vi "CFG Parse Registry Instructions.vi"(0 "Special Instructions":string, 1 "Section":string) -> (4 "Subkey":string, 8 "Registry Item":bool)   [LabVIEW 2012]
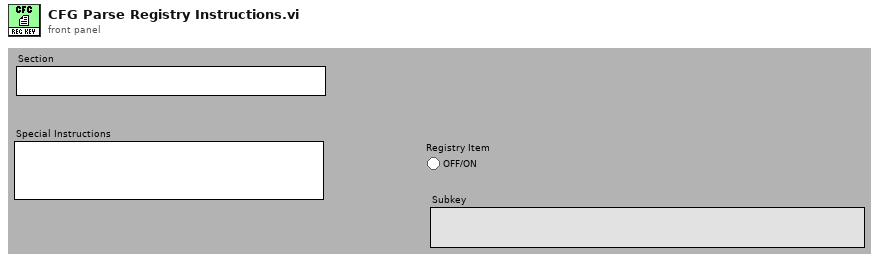
[diagram p1: front panel]
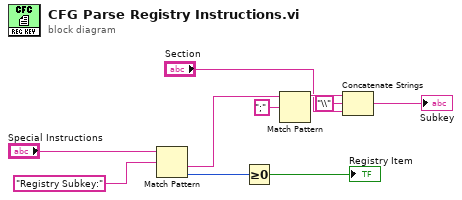
[diagram p0: block diagram]
diagram:
  n1 = Match Pattern(string="Special Instructions", regular expression="Registry Subkey:") -> (after substring=w6:string, offset past match=w9:i32)  [unwired: 3 out]
  n2 = Greater Or Equal To 0?(x=w9) -> (x >= 0?=→"Registry Item":bool)
  n3 = Match Pattern(string=w6, regular expression=";") -> (before substring=w4:string)  [unwired: 4 out]
  n4 = Concatenate Strings(w4, "\\" ("string"), "Section") -> (→"Subkey":string)
